vi "Framework_Initialize.vi"(8 "error in (no error)":errorcluster, 11 "Class in":refnum<class "IB_MSI.lvclass">) -> (0 "error out":errorcluster, 1 "helpTopics":string[](array[string]), 2 "pageTitles":string[](array[string]), 3 "Class out":refnum<class "IB_MSI.lvclass">, 4 "helpFile":string, 5 "pages":path[](array[path]))   [LabVIEW 2020, in "IB_MSI.lvclass"]
uses:
  <vilib>/AppBuilder/IB_Classes/MSI/IB_MSI.lvclass
  <vilib>/AppBuilder/IB_Classes/MSI/IB_MSI.lvclass/IB_MSI.ctl
panel:
  in  "pageTitles_MSI":string[](array[string])=["Product Information", "Destinations", "Source Files", "Source File Settings", "Shortcuts", "Additional Installers", "Dialog Information", "Registry", "Hardware Configuration", "Version Information", "Web Services", "Windows Security", "Advanced"]
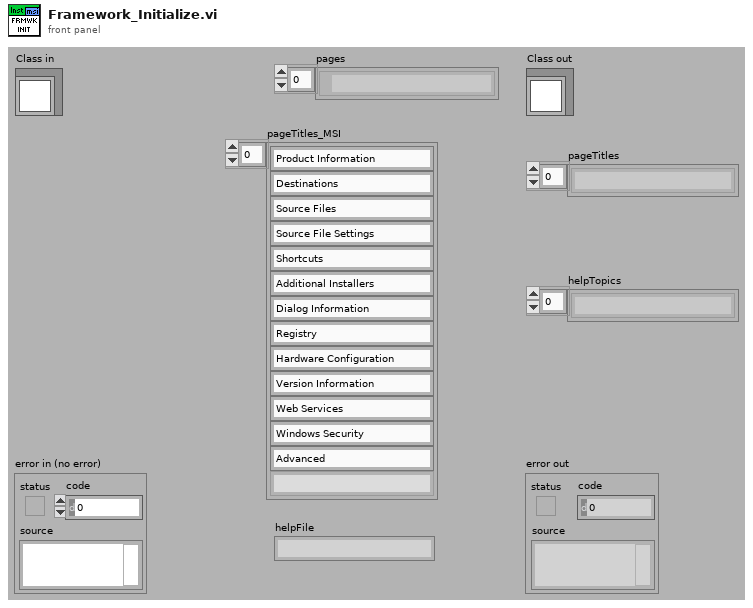
[diagram p1: front panel]
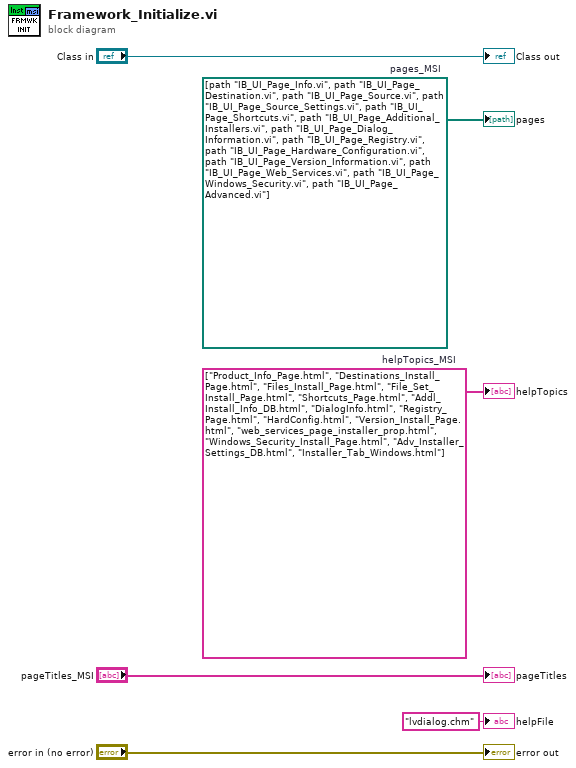
[diagram p0: block diagram]
diagram:
  w2 = path[] [path "IB_UI_Page_Info.vi", path "IB_UI_Page_Destination.vi", path "IB_UI_Page_Source.vi", path "IB_UI_Page_Source_Settings.vi", path "IB_UI_Page_Shortcuts.vi", path "IB_UI_Page_Additional_Installers.vi", path "IB_UI_Page_Dialog_Information.vi", path "IB_UI_Page_Registry.vi", path "IB_UI_Page_Hardware_Configuration.vi", path "IB_UI_Page_Version_Information.vi", path "IB_UI_Page_Web_Services.vi", path "IB_UI_Page_Windows_Security.vi", path "IB_UI_Page_Advanced.vi"]  # pages_MSI
  w3 = string[] ["Product_Info_Page.html", "Destinations_Install_Page.html", "Files_Install_Page.html", "File_Set_Install_Page.html", "Shortcuts_Page.html", "Addl_Install_Info_DB.html", "DialogInfo.html", "Registry_Page.html", "HardConfig.html", "Version_Install_Page.html", "web_services_page_installer_prop.html", "Windows_Security_Install_Page.html", "Adv_Installer_Settings_DB.html", "Installer_Tab_Windows.html"]  # helpTopics_MSI
  "error out" <- "error in (no error)"
  "Class out" <- "Class in"
  "pages" <- w2
  "helpTopics" <- w3
  "pageTitles" <- "pageTitles_MSI"
  "helpFile" <- "lvdialog.chm" ("helpFile")
